vi "Calc - C.vi"(7 "DO":dbl, 10 "P1":dbl, 11 "Temps.01-00-9213":dbl[](array[numeric])) -> (3 "C":dbl)   [LabVIEW 2018, in "Controller (Host).lvlib"]
uses:
  Controller (Host).lvlib
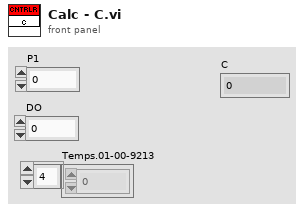
[diagram p1: front panel]
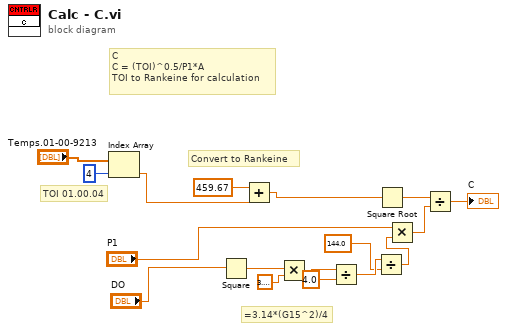
[diagram p0: block diagram]
diagram:
  # "TOI 01.00.04"
  # "C \nC = (TOI)^0.5/P1*A\nTOI to Rankeine for calculation"
  # "Convert to Rankeine"
  # "=3.14*(G15^2)/4"
  n1 = Index Array(array="Temps.01-00-9213", index=4) -> (element=w1:dbl)
  n2 = Square(x="DO") -> (x^2=w16:dbl)
  n3 = Add(x=459.67, y=w1) -> (x+y=w11:dbl)
  n4 = Multiply(x=w16, y=3.141592653589793) -> (x*y=w15:dbl)
  n5 = Divide(x=w15, y=4.0) -> (x/y=w9:dbl)
  n6 = Divide(x=w9, y=144.0 ("x")) -> (x/y=w7:dbl)
  n7 = Square Root(x=w11) -> (sqrt(x)=w13:dbl)
  n8 = Multiply(x="P1", y=w7) -> (x*y=w12:dbl)
  n9 = Divide(x=w13, y=w12) -> (x/y=→"C":dbl)
